vi "Facade.vi"(0 "Data In":T8, 2 "Display State In":T2={"Nspeakers"=0, "actions"=[], "Wspeaker"=13, "Wmic"=13, "sel mic"=13, "hover"={"type"=enum."None", "index"=0}, "locked"=FALSE, "states"=[], "sel speak"=13, "selected"=refnum, "Events"={"Mic change"=refnum, "Selection change"=refnum}}, 3 "Container State":T7) -> (6 "Data Out":T8, 7 "Display State Out":T2={"Nspeakers"=0, "actions"=[], "Wspeaker"=13, "Wmic"=13, "sel mic"=13, "hover"={"type"=enum."None", "index"=0}, "locked"=FALSE, "states"=[], "sel speak"=13, "selected"=refnum, "Events"={"Mic change"=refnum, "Selection change"=refnum}}, 8 "Action":T1)   [LabVIEW 2015, in "HRTF Config.xctl"]
uses:
  HRTF Config.xctl
  Data.vi
  <vilib>/_xctls/Container State.ctl
  State.vi
  Hover Data.ctl
  Hover Item.ctl
  Speaker State.ctl
  Events.ctl
  Selection changed.ctl
  <vilib>/_xctls/Action.ctl
  <vilib>/_xctls/XControlSupport.lvlib
panel:
  out "angle":string
  out "selected":picture
  out "mics":picture
  out "speakers":picture
  out "back":picture
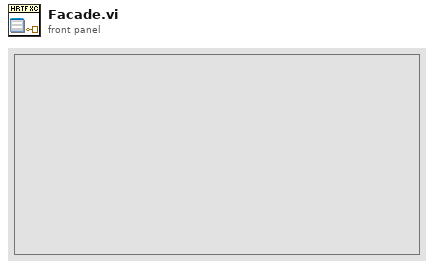
[diagram p1: front panel]
types:
  T1 = typedef "XControlSupport.lvlib/Action.ctl" = cluster{"Data Changed?":bool, "State Changed?":bool, "Action Name":string}
  T2 = typedef "HRTF Config.xctl/State.vi" = cluster{"Nspeakers":i32, "actions":string[], "Wspeaker":i32, "Wmic":i32, "sel mic":i32, "hover":T3, "locked":bool, "states":T5[], "sel speak":i32, "selected":refnum<vi>, "Events":T6}
  T3 = typedef "HRTF Config.xctl/Hover Data.ctl" = cluster{"type":T4, "index":i32}
  T4 = typedef "HRTF Config.xctl/Hover Item.ctl" = enum16{"None", "Speaker", "Mic"}
  T5 = typedef "HRTF Config.xctl/Speaker State.ctl" = cluster{"right cal":bool, "left cal":bool, "selected":bool}
  T6 = typedef "HRTF Config.xctl/Events.ctl" = cluster{"Mic change":refnum<user-event>, "Selection change":refnum<user-event>}
  T7 = typedef "XControlSupport.lvlib/Container State.ctl" = cluster{"Indicator?":bool, "Run Mode?":bool, " Refnum":refnum<vi>}
  T8 = typedef "HRTF Config.xctl/Data.vi" = i32
  T9 = typedef "LVPoint32TypeDef.ctl" = cluster{"Horizontal":i32, "Vertical":i32}
  T10 = cluster{"Min Control Width":i32, "Min Control Height":i32}
  T11 = typedef "LVPointTypeDef.ctl" = cluster{"Horizontal":i16, "Vertical":i16}
  T12 = typedef "HRTF Config.xctl/Layout.ctl" = cluster{"origin":cluster{"X":i32, "Y":i32}, "Items":T13[], "ring diameter":i32, "mics":cluster{"X":i32, "Y":i32}[]}
  T13 = typedef "HRTF Config.xctl/Item.ctl" = cluster{"center":cluster{"X":i32, "Y":i32}, "angle":dbl}
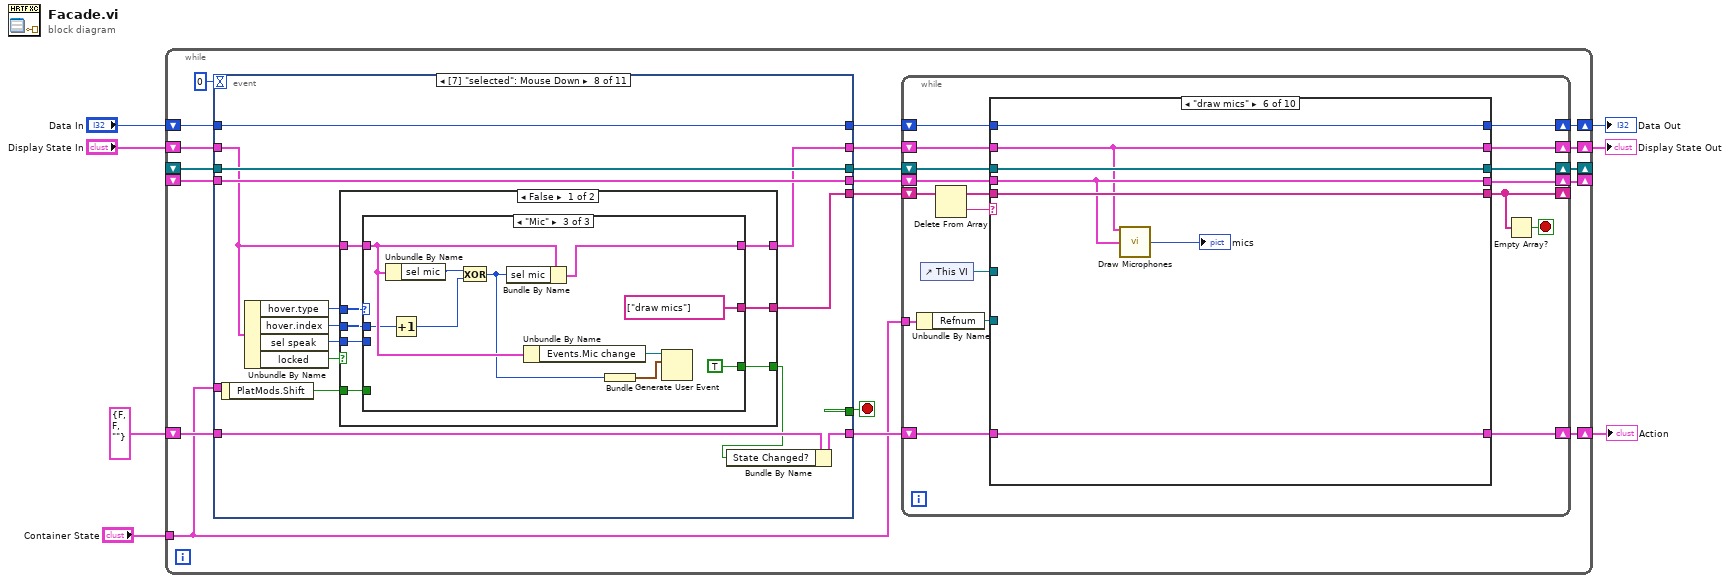
[diagram p0: block diagram]
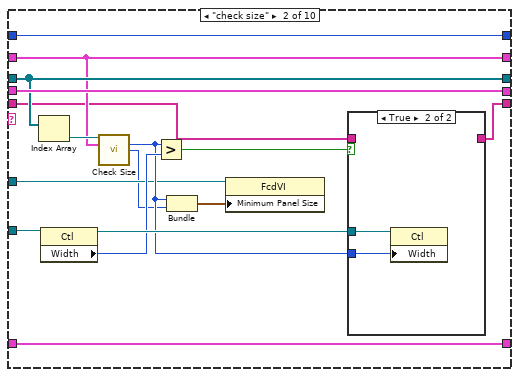
[diagram p3: hidden frame]
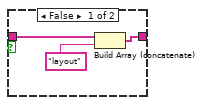
[diagram p4: hidden frame]
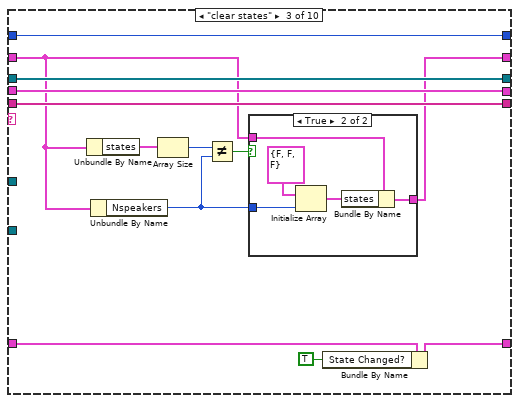
[diagram p5: hidden frame]
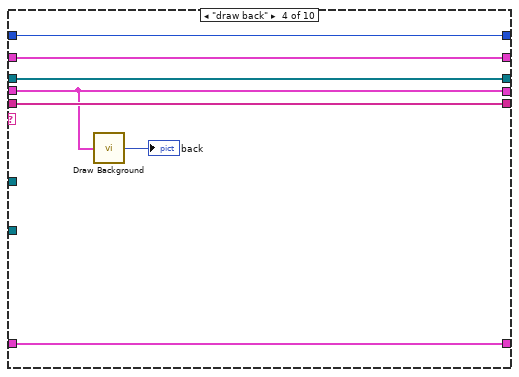
[diagram p7: hidden frame]
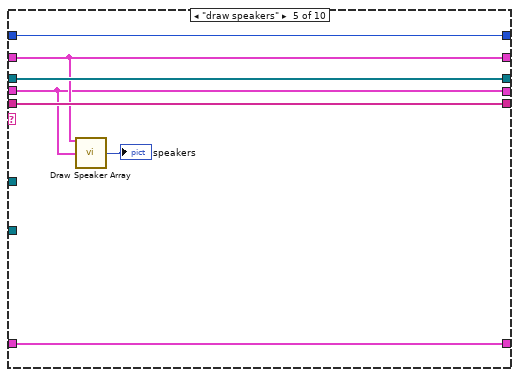
[diagram p8: hidden frame]
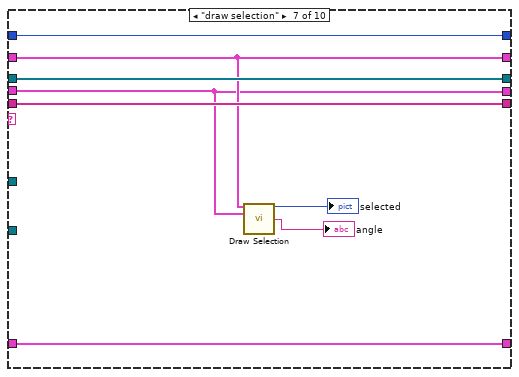
[diagram p9: hidden frame]
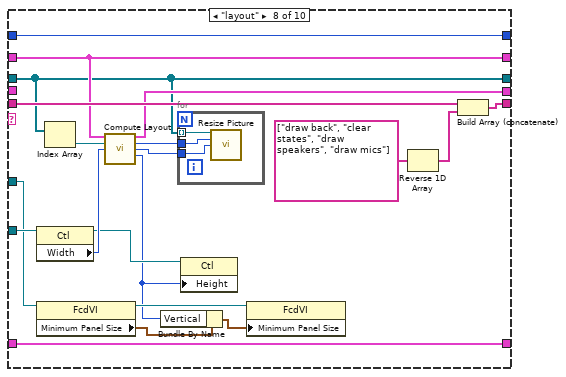
[diagram p10: hidden frame]
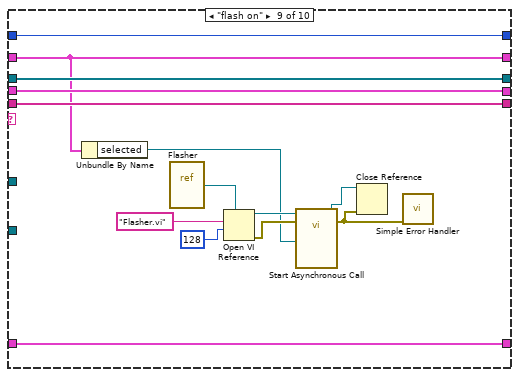
[diagram p11: hidden frame]
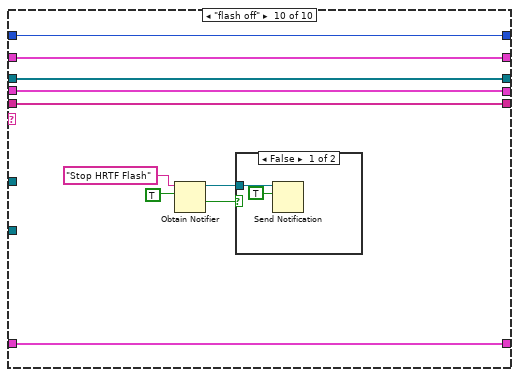
[diagram p12: hidden frame]
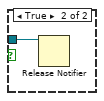
[diagram p13: hidden frame]
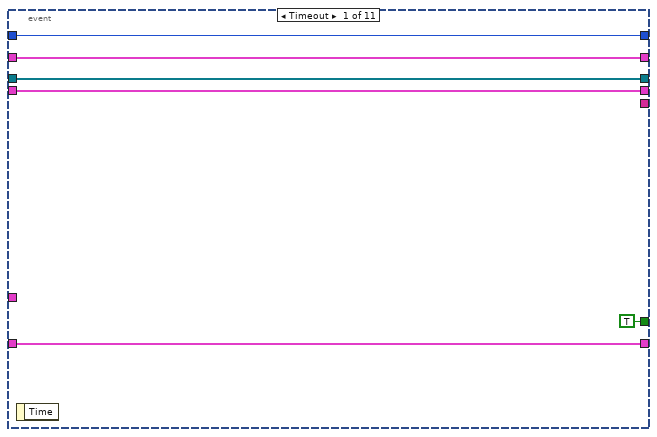
[diagram p14: hidden frame]
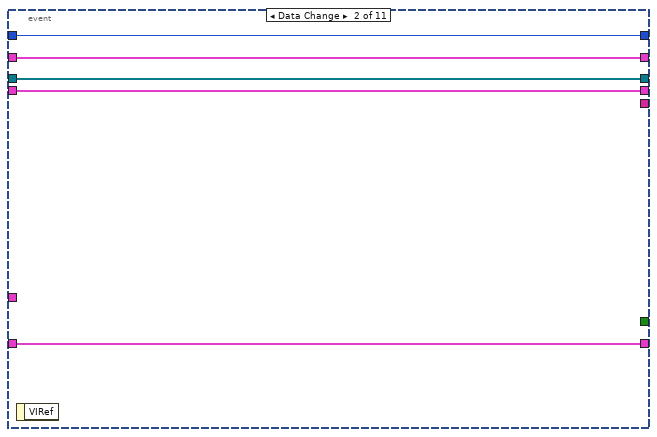
[diagram p15: hidden frame]
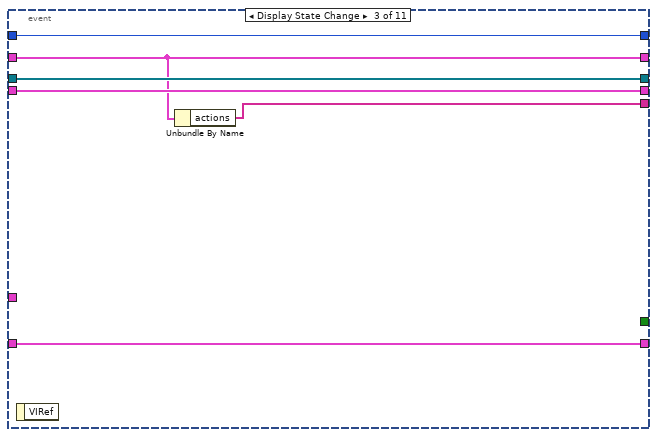
[diagram p16: hidden frame]
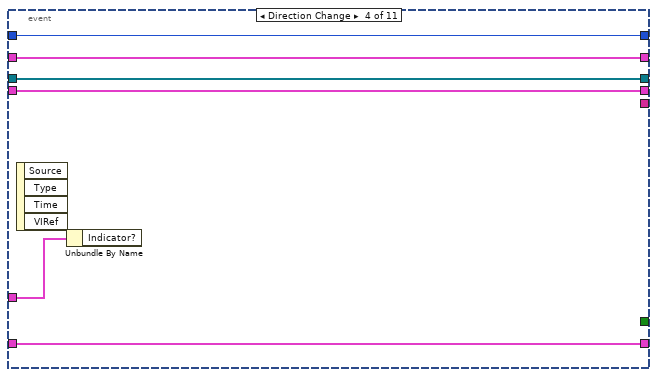
[diagram p17: hidden frame]
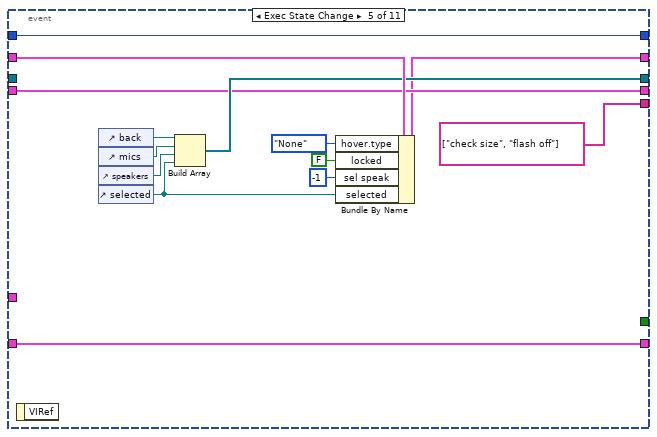
[diagram p18: hidden frame]
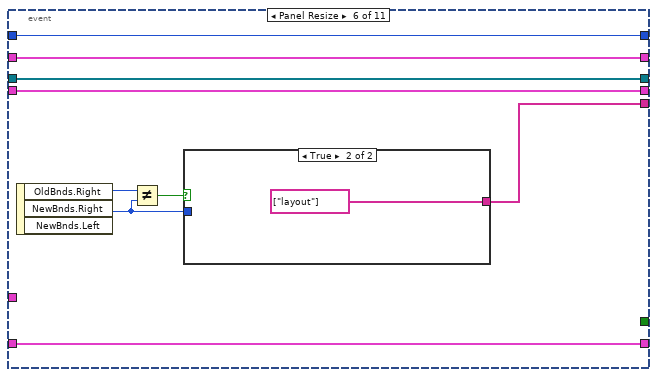
[diagram p19: hidden frame]
diagram:
  n1 = while {
    shift-right: [w15] -> w4
    shift-left: "Display State In" -> [w26]
    tunnel: "Container State" -> [w11]
    shift-right: [w16] -> w7
    shift-left: "Data In" -> [w23]
    shift-right: [w13] -> w2
    shift-left: T1 {"Data Changed?"=FALSE, "State Changed?"=FALSE, "Action Name"=""} ("Action") -> [w22]
    shift-right: [w14] -> _
    shift-left: _ -> [w21]
    shift-right: [w10] -> _
    shift-left: _ -> [w9]
    stop <- w25 stop-if-true
    n2 = event shown="[7] \"selected\": Mouse Down" {
      selector: _ -> [_ _ _ _ _ _ _ _ _ _ _]
      dyn-events: _ -> [_ _ _ _ _ _ _ _ _ _ _]
      timeout: 0 -> [_ _ _ _ _ _ _ _ _ _ _]
      tunnel: w26 -> [w173 w179 w181 w191 w201 w215 w218 w254 w304 w317 w323]
      tunnel: [w173 w179 w181 w191 w197 w215 w222 w253 w303 w317 w328] -> w18
      tunnel: [TRUE _ _ _ _ _ _ _ _ _ _] -> w25
      tunnel: w11 -> [_ _ _ w192 _ _ _ _ _ _ _]
      tunnel: w23 -> [w172 w180 w186 w190 w206 w214 w227 w260 w308 w321 w337]
      tunnel: [w172 w180 w186 w190 w206 w214 w227 w260 w308 w321 w337] -> w17
      tunnel: [w174 w178 w185 w189 w205 w213 w221 w252 w302 w320 w332] -> w12
      tunnel: w22 -> [w174 w178 w185 w189 w205 w213 w226 w259 w307 w320 w336]
      tunnel: [w171 w177 w184 w188 w200 w212 w225 w258 w306 w319 w335] -> w19
      tunnel: w21 -> [w171 w177 w184 w188 _ w212 w225 w258 w306 w319 w335]
      tunnel: [_ _ w182 _ string[] ["check size", "flash off"] w207 w219 w250 w300 _ string[] ["draw selection", "draw speakers"] ("String")] -> w20
      tunnel: w9 -> [w170 w176 w183 w187 w198 w208 w223 w256 w305 w318 w334]
      tunnel: [w170 w176 w183 w187 w198 w208 w223 w256 w305 w318 w334] -> w8
      event Timeout {
        n3 = event-data() -> ()  [unwired: 1 in, 1 out]
      }
      event Data Change {
        n4 = event-data() -> ()  [unwired: 1 in, 1 out]
      }
      event Display State Change {
        n5 = event-data() -> ()  [unwired: 1 in, 1 out]
        n6 = Unbundle By Name(w181) -> ("actions"=w182:string[])
      }
      event Direction Change {
        n7 = event-data() -> ()  [unwired: 1 in, 4 out]
        n8 = Unbundle By Name(w192) -> ()  [unwired: 1 out]
      }
      event Exec State Change {
        n9 = event-data() -> ()  [unwired: 1 in, 1 out]
        n10 = control-ref of="back"() -> (w202:refnum<vi>)
        n11 = control-ref of="mics"() -> (w203:refnum<vi>)
        n12 = control-ref of="speakers"() -> (w204:refnum<vi>)
        n13 = control-ref of="selected"() -> (w193:refnum<vi>)
        n14 = Build Array(w202, w203, w204, w193) -> (w200:refnum<vi>[])
        n15 = Bundle By Name(cluster=w201, "hover.type"=Hover_Item."None", "locked"=FALSE, "sel speak"=-1, "selected"=w193) -> (w197:T2)
      }
      event Panel Resize {
        n16 = event-data() -> ("OldBnds.Right"=w211:i16, "NewBnds.Right"=w210:i16)  [unwired: 1 in, 1 out]
        n17 = Not Equal?(x=w211, y=w210) -> (x != y?=w209:bool)
        n18 = case shown="True" w209 {
          tunnel: w210 -> [_ _]
          tunnel: [_ string[] ["layout"] ("String")] -> w207
          frame False {
          }
          frame True {
          }
        }
      }
      event "selected": Mouse Move {
        n19 = event-data() -> ("Coords"=w224:T9)  [unwired: 1 in]
        n20 = Unbundle By Name(w218) -> ("locked"=w217:bool)
        n21 = case shown="False" w217 {
          tunnel: w224 -> [w240 _]
          tunnel: w223 -> [w239 _]
          tunnel: [w231 w246] -> w222
          tunnel: [w230 _] -> w220
          tunnel: [w229 _] -> w219
          tunnel: w218 -> [w228 w246]
          frame False {
            n22 = call "Process Mouse Move.vi"("State"=w228, "Layout"=w239, "Coords"=w240) -> ("Hover Data"=w232:T3)  [unwired: 12 in]
            n23 = Unbundle By Name(w228) -> ("hover.type"=w237:T4, "hover.index"=w234:i32)
            n24 = Unbundle By Name(w232) -> ("type"=w238:T4, "index"=w235:i32)
            n25 = Not Equal?(x=w237, y=w238) -> (x != y?=w236:bool)
            n26 = Not Equal?(x=w235, y=w234) -> (x != y?=w233:bool)
            n27 = Or(x=w236, y=w233) -> (x .or. y?=w230:bool)
            n28 = case shown="True" w230 {
              tunnel: w232 -> [_ w243]
              tunnel: w228 -> [w241 w245]
              tunnel: [w241 w244] -> w231
              tunnel: [_ string[] ["draw selection"] ("String")] -> w229
              frame False {
              }
              frame True {
                n29 = Bundle By Name(cluster=w245, "hover"=w243) -> (w244:T2)
              }
            }
          }
          frame True {
          }
        }
        n30 = Bundle By Name(cluster=w226, "State Changed?"=w220) -> (w221:T1)
      }
      event "selected": Mouse Down {
        n31 = event-data() -> ("PlatMods.Shift"=w247:bool)  [unwired: 1 in]
        n32 = Unbundle By Name(w254) -> ("hover.type"=w257:T4, "hover.index"=w255:i32, "sel speak"=w248:i32, "locked"=w249:bool)
        n33 = case shown="False" w249 {
          tunnel: w257 -> [w268 _]
          tunnel: w255 -> [w267 _]
          tunnel: w254 -> [w266 w298]
          tunnel: [w265 w298] -> w253
          tunnel: [w264 _] -> w251
          tunnel: [w263 _] -> w250
          tunnel: w248 -> [w262 _]
          tunnel: w247 -> [w261 _]
          frame False {
            n34 = case shown="\"Mic\"" w268 {
              tunnel: w266 -> [w272 w275 w292]
              tunnel: w267 -> [_ w278 w290]
              tunnel: [w270 w282 w296] -> w265
              tunnel: [TRUE TRUE TRUE] -> w264
              tunnel: [_ string[] ["draw selection", "draw speakers"] ("String") string[] ["draw mics"] ("String")] -> w263
              tunnel: w262 -> [_ w281 _]
              tunnel: w261 -> [_ w280 _]
              frame "None", Default {
                n35 = Bundle By Name(cluster=w272, "sel speak"=-1) -> (w270:T2)
              }
              frame "Speaker" {
                n36 = Unbundle By Name(w275) -> ("Events.Selection change"=w277:refnum<user-event>)
                n37 = Unbundle By Name(w275) -> ("states"=w284:T5[])
                n38 = call "Update Speaker Selection.vi"("states in"=w284, "index"=w278, "sel speak"=w281, "Shift"=w280) -> ("states out"=w274:T5[])  [unwired: 11 in]
                n39 = Bundle By Name(cluster=w275, "states"=w274, "sel speak"=w278) -> (w282:T2)
                n40 = for {
                  tunnel: w274 -> [w287] mode=indexing
                  tunnel: [w285] -> w273 mode=indexing if=w286
                  i -> [w285]
                  n41 = Unbundle By Name(w287) -> ("selected"=w286:bool)
                }
                n42 = Bundle(w273) -> (w276:cluster{i32[]})  [unwired: 1 in]
                n43 = Generate User Event(user event=w277, event data cluster=w276) -> ()  [unwired: 2 in, 2 out]
              }
              frame "Mic" {
                n44 = Unbundle By Name(w292) -> ("sel mic"=w291:i32)
                n45 = Increment(x=w290) -> (x+1=w288:i32)
                n46 = Exclusive Or(1:w288, 2:w291) -> (0:w289:i32)
                n47 = Bundle By Name(cluster=w292, "sel mic"=w289) -> (w296:T2)
                n48 = Unbundle By Name(w292) -> ("Events.Mic change"=w294:refnum<user-event>)
                n49 = Bundle(w289) -> (w293:cluster{i32})  [unwired: 1 in]
                n50 = Generate User Event(user event=w294, event data cluster=w293) -> ()  [unwired: 2 in, 2 out]
              }
            }
          }
          frame True {
          }
        }
        n51 = Bundle By Name(cluster=w259, "State Changed?"=w251) -> (w252:T1)
      }
      event Mouse Leave {
        n52 = event-data() -> ()  [unwired: 1 in, 1 out]
        n53 = Unbundle By Name(w304) -> ("locked"=w299:bool)
        n54 = case shown="False" w299 {
          tunnel: w304 -> [w314 w315]
          tunnel: [w313 w315] -> w303
          tunnel: [TRUE _] -> w301
          tunnel: [string[] ["draw selection"] ("String") _] -> w300
          frame False {
            n55 = Bundle By Name(cluster=w314, "sel speak"=-1, "hover.type"=Hover_Item."None") -> (w313:T2)
          }
          frame True {
          }
        }
        n56 = Bundle By Name(cluster=w307, "State Changed?"=w301) -> (w302:T1)
      }
      event "selected": Shortcut Menu Activation? {
        n57 = event-data() -> ()  [unwired: 1 in, 1 out]
        n58 = Unbundle By Name(w317) -> ("locked"=w316:bool)
        n59 = event-data("Discard?"=w316) -> ()  [unwired: 1 in, 1 out]
      }
      event "selected": Shortcut Menu Selection (User) {
        n60 = event-data() -> ("ItemTag"=w330:string)  [unwired: 1 in]
        n61 = Unbundle By Name(w323) -> ("states"=w333:T5[])
        n62 = Unbundle By Name(w323) -> ("sel mic"=w329:i32)
        n63 = for {
          tunnel: w333 -> [w341] mode=indexing
          tunnel: w329 -> [w348]
          tunnel: w330 -> [w344]
          tunnel: [w342] -> w327 mode=indexing
          tunnel: [w339] -> w324 mode=indexing if=w338
          i -> [w339]
          n64 = Equal To 0?(x=w348) -> (x = 0?=w347:bool)
          n65 = Unbundle By Name(w341) -> ("right cal"=w346:bool, "left cal"=w345:bool)
          n66 = Unbundle By Name(w341) -> ("selected"=w340:bool)
          n67 = Select(t=w346, s=w347, f=w345) -> (s? t:f=w343:bool)
          n68 = case shown="\"cmClearAll\"" w344 {
            tunnel: w343 -> [_ _ w352 _ w357]
            tunnel: [FALSE TRUE w351 FALSE w354] -> w338
            tunnel: w340 -> [_ _ _ _ w355]
            frame "False", Default {
            }
            frame "cmSelectAll" {
            }
            frame "cmSelectIncomplete" {
              n69 = Not(x=w352) -> (.not. x?=w351:bool)
            }
            frame "cmClearAll" {
            }
            frame "cmClearComplete" {
              n70 = Not(x=w357) -> (.not. x?=w356:bool)
              n71 = And(x=w356, y=w355) -> (x .and. y?=w354:bool)
            }
          }
          n72 = Bundle By Name(cluster=w341, "selected"=w338) -> (w342:T5)
        }
        n73 = Unbundle By Name(w323) -> ("Events.Selection change"=w322:refnum<user-event>)
        n74 = Bundle By Name(cluster=w336, "State Changed?"=TRUE) -> (w332:T1)
        n75 = Bundle By Name(cluster=w323, "states"=w327) -> (w328:T2)
        n76 = Bundle(w324) -> (w325:cluster{i32[]})  [unwired: 1 in]
        n77 = Generate User Event(user event=w322, event data cluster=w325) -> ()  [unwired: 2 in, 2 out]
      }
    }
    n78 = while {
      shift-right: [w39] -> w16
      shift-left: w17 -> [w43]
      shift-right: [w38] -> w15
      shift-left: w18 -> [w42]
      shift-right: [w37] -> w14
      shift-left: w19 -> [w41]
      shift-right: [w35] -> w13
      shift-left: w12 -> [w40]
      shift-right: [w36] -> _
      shift-left: w20 -> [w34]
      tunnel: w11 -> [w28]
      shift-right: [w30] -> w10
      shift-left: w8 -> [w29]
      stop <- w44 stop-if-true
      n79 = Unbundle By Name(w28) -> ("Refnum"=w27:refnum<vi>)
      n80 = control-ref of="This VI"() -> (w31:refnum<vi>)
      n81 = Delete From Array(array=w34) -> (deleted portion=w32:string, array with subset deleted=w33:string[])  [unwired: 2 in]
      n82 = case shown="\"draw mics\"" w32 {
        tunnel: w43 -> [w50 w66 w84 w97 w104 w111 w119 w139 w156 w166]
        tunnel: w42 -> [w49 w61 w76 w96 w100 w106 w115 w136 w151 w165]
        tunnel: w41 -> [w48 w63 w83 w95 w103 w110 w118 w129 w155 w164]
        tunnel: w33 -> [w47 w56 w82 w94 w102 w109 w117 w138 w154 w163]
        tunnel: w40 -> [w46 w65 w81 w93 w101 w108 w116 w137 w153 w162]
        tunnel: [w50 w66 w84 w97 w104 w111 w119 w139 w156 w166] -> w39
        tunnel: [w49 w61 w79 w96 w100 w106 w115 w136 w151 w165] -> w38
        tunnel: [w48 w63 w83 w95 w103 w110 w118 w129 w155 w164] -> w37
        tunnel: [w47 w55 w82 w94 w102 w109 w117 w134 w154 w163] -> w36
        tunnel: [w46 w65 w78 w93 w101 w108 w116 w137 w153 w162] -> w35
        tunnel: w31 -> [_ w53 _ _ _ _ _ w125 _ _]
        tunnel: [w45 w64 w80 w92 w99 w107 w114 w132 w152 w161] -> w30
        tunnel: w29 -> [w45 w64 w80 w92 w99 w107 w114 _ w152 w161]
        tunnel: w27 -> [_ w60 _ _ _ _ _ w135 _ _]
        frame "False", Default {
        }
        frame "check size" {
          n83 = Index Array(array=w63) -> (element=w62:refnum<vi>)  [unwired: 1 in]
          n84 = property class="Ctl"(reference=w60) -> (reference out=w59:refnum<vi>, "Width"=w58:u32)  [unwired: 1 in, 1 out]
          n85 = call "Check Size.vi"("picture ref"=w62, "State"=w61) -> ("Min Control Width"=w54:i32, "Min Control Height"=w51:i32)  [unwired: 12 in]
          n86 = Greater?(x=w54, y=w58) -> (0:w57:bool)
          n87 = Bundle("Min Control Width"=w54, "Min Control Height"=w51) -> (w52:T10)  [unwired: 1 in]
          n88 = property class="FcdVI"(reference=w53, "Minimum Panel Size"=w52) -> ()  [unwired: 1 in, 2 out]
          n89 = case shown="True" w57 {
            tunnel: w59 -> [_ w71]
            tunnel: w54 -> [_ w70]
            tunnel: w56 -> [w69 _]
            tunnel: [w68 _] -> w55
            frame False {
              n90 = Build Array (concatenate)(w69, "layout" ("String")) -> (w68:string[])
            }
            frame True {
              n91 = property class="Ctl"(reference=w71, "Width"=w70) -> ()  [unwired: 1 in, 2 out]
            }
          }
        }
        frame "clear states" {
          n92 = Unbundle By Name(w76) -> ("states"=w75:T5[])
          n93 = Unbundle By Name(w76) -> ("Nspeakers"=w73:i32)
          n94 = Array Size(array=w75) -> (size(s)=w74:i32)
          n95 = Not Equal?(x=w74, y=w73) -> (x != y?=w72:bool)
          n96 = case shown="True" w72 {
            tunnel: w73 -> [_ w90]
            tunnel: [w85 w87] -> w79
            tunnel: w76 -> [w85 w86]
            frame False {
            }
            frame True {
              n97 = Initialize Array(T5 {"right cal"=FALSE, "left cal"=FALSE, "selected"=FALSE} ("Speaker State"), w90) -> (w88:T5[])
              n98 = Bundle By Name(cluster=w86, "states"=w88) -> (w87:T2)
            }
          }
          n99 = Bundle By Name(cluster=w81, "State Changed?"=TRUE) -> (w78:T1)
        }
        frame "draw back" {
          n100 = call "Draw Background.vi"("Layout"=w92) -> ("2D Picture"=→"back":picture)  [unwired: 14 in]
        }
        frame "draw speakers" {
          n101 = call "Draw Speaker Array.vi"("State"=w100, "Layout"=w99) -> ("2D Picture"=→"speakers":picture)  [unwired: 13 in]
        }
        frame "draw mics" {
          n102 = call "Draw Microphones.vi"("State"=w106, "Layout"=w107) -> ("2D Picture"=→"mics":picture)  [unwired: 13 in]
        }
        frame "draw selection" {
          n103 = call "Draw Selection.vi"("Display State In"=w115, "Layout"=w114) -> ("empty picture"=→"selected":picture, "String"=→"angle":string)  [unwired: 12 in]
        }
        frame "layout" {
          n104 = property class="Ctl"(reference=w135) -> (reference out=w126:refnum<vi>, "Width"=w131:u32)  [unwired: 1 in, 1 out]
          n105 = property class="FcdVI"(reference=w125) -> (reference out=w124:refnum<vi>, "Minimum Panel Size"=w123:T11)  [unwired: 1 in, 1 out]
          n106 = Index Array(array=w129) -> (element=w130:refnum<vi>)  [unwired: 1 in]
          n107 = call "Compute Layout.vi"("State"=w136, "picture ref"=w130, "Size"=w131) -> ("Layout"=w132:T12, "Wpict"=w128:u32, "Hpict"=w127:u32, "Hcontrol"=w121:u32)  [unwired: 9 in]
          n108 = Bundle By Name(cluster=w123, "Vertical"=w121) -> (w122:T11)
          n109 = for {
            tunnel: w129 -> [w142] mode=indexing
            tunnel: w128 -> [w141]
            tunnel: w127 -> [w140]
            n110 = call "Resize Picture.vi"("Picture ref"=w142, "new width"=w141, "new height"=w140) -> ()  [unwired: 13 in]
          }
          n111 = property class="Ctl"(reference=w126, "Height"=w121) -> ()  [unwired: 1 in, 2 out]
          n112 = property class="FcdVI"(reference=w124, "Minimum Panel Size"=w122) -> ()  [unwired: 1 in, 2 out]
          n113 = Reverse 1D Array(array=string[] ["draw back", "clear states", "draw speakers", "draw mics"]) -> (reversed array=w120:string[])
          n114 = Build Array (concatenate)(w138, w120) -> (w134:string[])
        }
        frame "flash on" {
          n115 = Unbundle By Name(w151) -> ("selected"=w143:refnum<vi>)
          n116 = vi-ref "Flasher.vi"() -> (w148:refnum<vi>)
          n117 = Open VI Reference(type specifier VI Refnum (for type only)=w148, vi path="Flasher.vi", options=128) -> (vi reference=w149:refnum<vi>, error out=w147:errorcluster)  [unwired: 3 in]
          n118 = call-by-ref "Start Asynchronous Call"(reference=w149, error in=w147, "reference"=w143) -> (reference out=w145:refnum<vi>, error out=w146:errorcluster)  [unwired: 15 in]
          n119 = Close Reference(reference=w145, error in (no error)=w146) -> ()  [unwired: 1 out]
          n120 = call <vilib>:"Simple Error Handler.vi"("error in (no error)"=w146) -> ()  [unwired: 4 in, 5 out]
        }
        frame "flash off" {
          n121 = Obtain Notifier(name (unnamed)="Stop HRTF Flash", notification data type=TRUE) -> (notifier out=w157:refnum<notifier>, created new?=w158:bool)  [unwired: 2 in, 1 out]
          n122 = case shown="False" w158 {
            tunnel: w157 -> [w168 w169]
            frame False {
              n123 = Send Notification(notification=TRUE, notifier=w168) -> ()  [unwired: 1 in, 2 out]
            }
            frame True {
              n124 = Release Notifier(notifier=w169) -> ()  [unwired: 2 in, 3 out]
            }
          }
        }
      }
      n125 = Empty Array?(array=w36) -> (empty?=w44:bool)
    }
  }
  "Display State Out" <- w4
  "Data Out" <- w7
  "Action" <- w2
